vi "Overlay Particle Analysis Results.vi"(6 "Color":u32(colorbox)=16711680, 7 "Group":string, 8 "error in":errorcluster, 9 "Overlay":enum16{"Bounding Box", "Center of Mass"}(ring), 10 "Particle Reports (Pixels)":T2(array[cluster]), 11 "Image":T1) -> (0 "error out":errorcluster, 3 "Image Out":T1)   [LabVIEW 2016]
doc: "Overlay targets at the location of the feature points in the specified colors."
uses:
  <vilib>/vision/Image Controls.llb/IMAQ Image.ctl
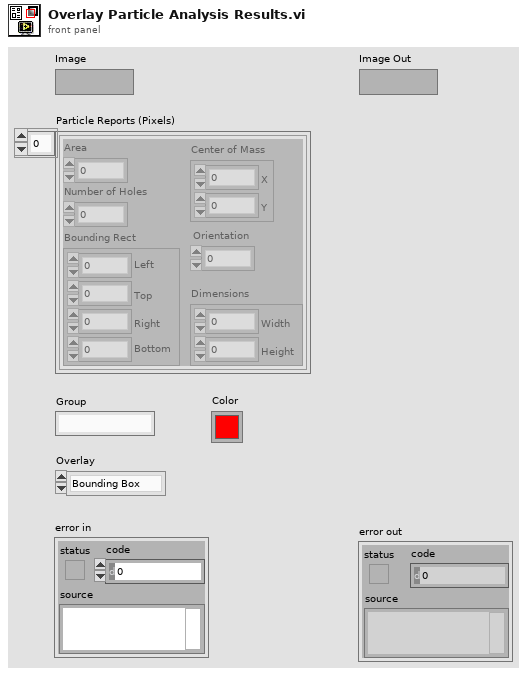
[diagram p1: front panel]
types:
  T1 = typedef "IMAQ Image.ctl" = refnum<image>
  T2 = cluster{"Area":dbl, "Number of Holes":dbl, "Bounding Rect":cluster{"Left":dbl, "Top":dbl, "Right":dbl, "Bottom":dbl}, "Center of Mass":cluster{"X":dbl, "Y":dbl}, "Orientation":dbl, "Dimensions":cluster{"Width":dbl, "Height":dbl}}[]
  T3 = cluster{"Left":dbl, "Top":dbl, "Right":dbl, "Bottom":dbl}
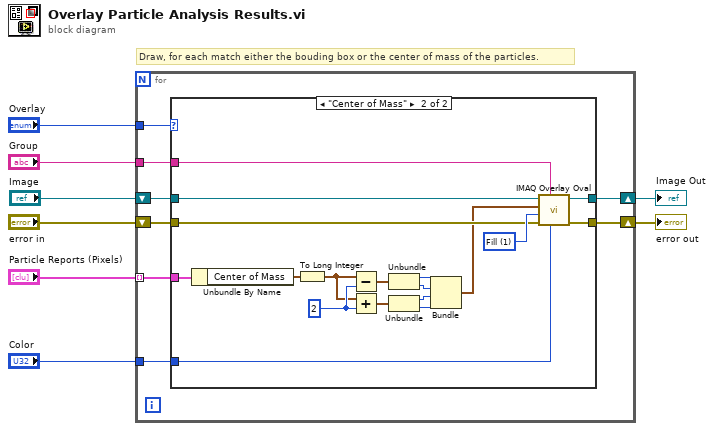
[diagram p0: block diagram]
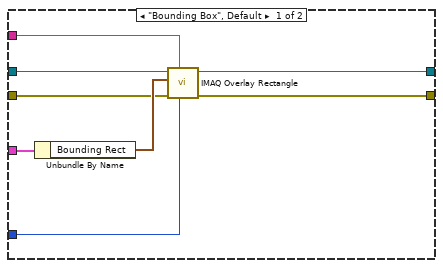
[diagram p2: hidden frame]
diagram:
  # "Draw, for each match either the bouding box or the center of mass of the particles."
  n1 = for {
    shift-right: [w9] -> w7
    shift-left: "Image" -> [w16]
    tunnel: "Particle Reports (Pixels)" -> [w14] mode=indexing
    tunnel: "Color" -> [w10]
    shift-right: [w11] -> w1
    shift-left: "error in" -> [w12]
    tunnel: "Overlay" -> [w15]
    tunnel: "Group" -> [w13]
    n2 = case shown="\"Center of Mass\"" w15 {
      tunnel: w16 -> [w24 w36]
      tunnel: w14 -> [w23 w34]
      tunnel: w13 -> [w21 w27]
      tunnel: w12 -> [w20 w35]
      tunnel: [w19 w29] -> w11
      tunnel: w10 -> [w18 w26]
      tunnel: [w17 w28] -> w9
      frame "Bounding Box", Default {
        n3 = Unbundle By Name(w23) -> ("Bounding Rect"=w22:T3)
        n4 = call "IMAQ Overlay Rectangle"("Color"=w18, "Group"=w21, "error in (no error)"=w20, "Rectangle"=w22, "Image"=w24) -> ("error out"=w19:errorcluster, "Image Out"=w17:T1)  [unwired: 5 in]
      }
      frame "Center of Mass" {
        w42 = u32 1 items=["Frame", "Fill"] ("Drawing Mode (Frame)")
        w37 = 2
        n5 = Unbundle By Name(w34) -> ("Center of Mass"=w31:cluster{"X":dbl, "Y":dbl})
        n6 = To Long Integer(number=w31) -> (32bit integer=w25:cluster{"X":i32, "Y":i32})
        n7 = Subtract(x=w25, y=w37) -> (x-y=w33:cluster{"X":i32, "Y":i32})
        n8 = Add(x=w25, y=w37) -> (x+y=w32:cluster{"X":i32, "Y":i32})
        n9 = Unbundle(w33) -> ("X"=w38:i32, "Y"=w39:i32)
        n10 = Unbundle(w32) -> ("X"=w40:i32, "Y"=w41:i32)
        n11 = Bundle("X"=w38, "Y"=w39, "X"=w40, "Y"=w41) -> (w30:cluster{"X":i32, "Y":i32, "X":i32, "Y":i32})  [unwired: 1 in]
        n12 = call "IMAQ Overlay Oval"("Color"=w26, "Group"=w27, "error in (no error)"=w35, "Drawing Mode (Frame)"=w42, "Bounding Rectangle"=w30, "Image"=w36) -> ("error out"=w29:errorcluster, "Image Out"=w28:T1)  [unwired: 4 in]
      }
    }
  }
  "Image Out" <- w7
  "error out" <- w1
